vi "Launch.vi"(9 "Alias":string, 10 "Actor":refnum<class "Actor.lvclass">) -> (0 "error out":errorcluster)   [LabVIEW 2021, in "jettl.lvlib" / "jettl.lvclass"]
uses:
  jettl.lvclass
  Actor/Actor.lvclass
  Create Top Level.vi
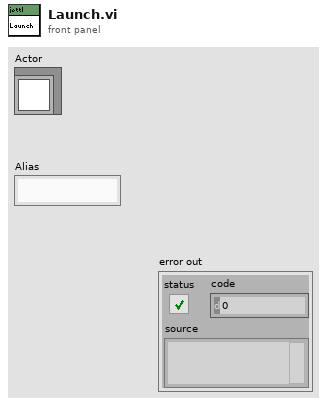
[diagram p1: front panel]
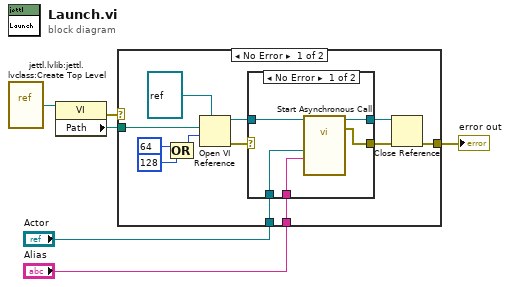
[diagram p0: block diagram]
diagram:
  n1 = vi-ref "jettl.lvlib:jettl.lvclass:Create Top Level.vi"() -> (w5:refnum<vi>)
  n2 = property class="VI"(reference=w5) -> (error out=w6:errorcluster, "Path"=w4:path)  [unwired: 1 in, 1 out]
  n3 = case shown="No Error" w6 {
    selector: w6 -> [_ w26]
    tunnel: [w16 w26] -> w1
    tunnel: w4 -> [w12 _]
    tunnel: "Alias" -> [w8 _]
    tunnel: "Actor" -> [w7 _]
    frame No Error {
      n4 = Compound Arithmetic op=OR(64 ("options: Multiple Clones,\n  Fire & Forget"), 128 ("options: Multiple Clones,\n  Fire & Forget")) -> (w14:i32)
      n5 = Open VI Reference(type specifier VI Refnum (for type only)=refnum<vi> refnum, vi path=w12, options=w14) -> (vi reference=w10:refnum<vi>, error out=w11:errorcluster)  [unwired: 3 in]
      n6 = case shown="No Error" w11 {
        selector: w11 -> [_ w25]
        tunnel: [w23 w24] -> w18
        tunnel: [w22 w25] -> w17
        tunnel: w10 -> [w21 w24]
        tunnel: w8 -> [w20 _]
        tunnel: w7 -> [w19 _]
        frame No Error {
          n7 = call-by-ref "Start Asynchronous Call"(reference=w21, "Alias"=w20, "Actor"=w19) -> (reference out=w23:refnum<vi>, error out=w22:errorcluster)  [unwired: 11 in]
        }
        frame Error {
        }
      }
      n8 = Close Reference(reference=w18, error in (no error)=w17) -> (error out=w16:errorcluster)
    }
    frame Error {
    }
  }
  "error out" <- w1
